vi "RT_TVA_2_boardcomp_DATA_vPXI.vi"(11 "TVA data":u8[](array[numeric])) -> (0 "TVA_Yaw [deg]":dbl, 1 "TVA_Pitch [deg]":dbl, 2 "Act 315 Angle \"Yaw\"":dbl(knob) scale=-3.0..3.0, 3 "Act 225 Angle \"Pitch\"":dbl(knob) scale=-3.0..3.0, 4 "CRC Check over Byte #10 to byte #84":bool, 5 "Control Variables (extra variables)":dbl[](array[numeric]), 6 "CRC Check over Byte #2 to Byte #7":bool)   [LabVIEW 2017]
panel:
  out "CRC data":u16 format="%x"
  out "CRC data comp":u16 format="%x"
  out "CRC addr":u16 format="%x"
  out "CRC addr comp":u16 format="%x"
  out "Roll DMARS [deg]":dbl
  out "Yaw DMARS [deg]":dbl
  out "Pitch DMARS [deg]":dbl
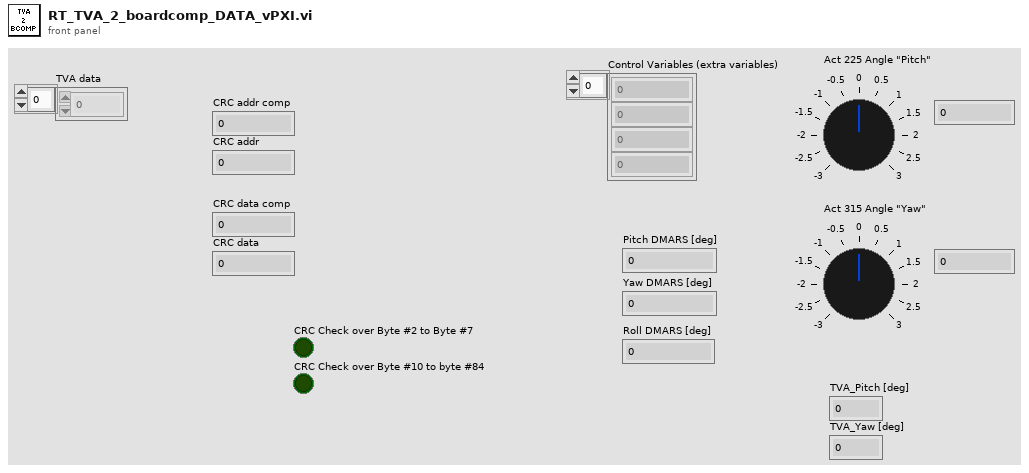
[diagram p1: front panel]
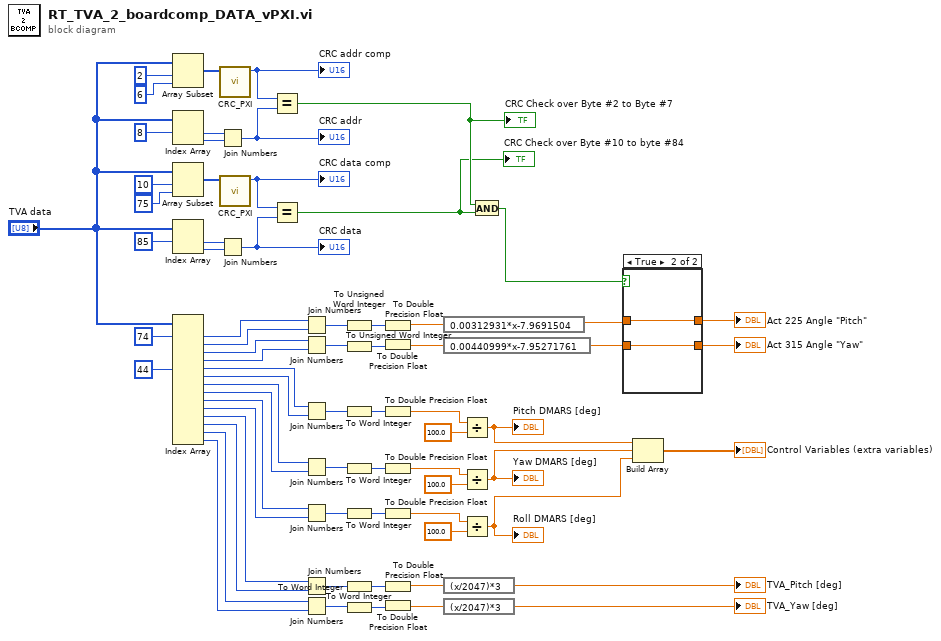
[diagram p0: block diagram]
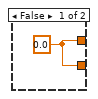
[diagram p2: hidden frame]
diagram:
  n1 = Array Subset(array="TVA data", index=2, length=6) -> (w37:u8[])
  n2 = Index Array(array="TVA data", index #1=8 ("index")) -> (element #1=w33:u8, element #2=w34:u8)  [unwired: 1 in]
  n3 = Array Subset(array="TVA data", index=10, length=75) -> (w27:u8[])
  n4 = Index Array(array="TVA data", index #1=85 ("index")) -> (element #1=w30:u8, element #2=w29:u8)  [unwired: 1 in]
  n5 = Index Array(array="TVA data", index #1=74 ("index"), index #5=44 ("index")) -> (element #1=w14:u8, element #2=w66:u8, element #3=w67:u8, element #4=w68:u8, element #5=w20:u8, element #6=w19:u8, element #7=w18:u8, element #8=w17:u8, element #9=w16:u8, element #10=w15:u8, element #11=w6:u8, element #12=w5:u8, element #13=w4:u8, element #14=w3:u8)  [unwired: 12 in]
  n6 = Join Numbers(hi=w33, lo=w34) -> ((hi.lo)=w32:u16)
  "CRC addr" <- w32
  n7 = Join Numbers(hi=w30, lo=w29) -> ((hi.lo)=w22:u16)
  "CRC data" <- w22
  n8 = call "CRC_PXI.vi"("Array"=w37) -> ("CRC"=w36:u16)  [unwired: 10 in]
  "CRC addr comp" <- w36
  n9 = call "CRC_PXI.vi"("Array"=w27) -> ("CRC"=w23:u16)  [unwired: 10 in]
  "CRC data comp" <- w23
  n10 = Equal?(x=w36, y=w32) -> (x = y?=w31:bool)
  "CRC Check over Byte #2 to Byte #7" <- w31
  n11 = Equal?(x=w23, y=w22) -> (x = y?=w24:bool)
  "CRC Check over Byte #10 to byte #84" <- w24
  n12 = Join Numbers(hi=w14, lo=w66) -> ((hi.lo)=w59:u16)
  n13 = Join Numbers(hi=w67, lo=w68) -> ((hi.lo)=w57:u16)
  n14 = Join Numbers(hi=w20, lo=w19) -> ((hi.lo)=w52:u16)
  n15 = Join Numbers(hi=w18, lo=w17) -> ((hi.lo)=w53:u16)
  n16 = Join Numbers(hi=w16, lo=w15) -> ((hi.lo)=w51:u16)
  n17 = Join Numbers(hi=w6, lo=w5) -> ((hi.lo)=w10:u16)
  n18 = Join Numbers(hi=w4, lo=w3) -> ((hi.lo)=w8:u16)
  n19 = To Unsigned Word Integer(number=w59) -> (unsigned 16bit integer=w58:u16)
  n20 = To Unsigned Word Integer(number=w57) -> (unsigned 16bit integer=w56:u16)
  n21 = To Word Integer(number=w52) -> (16bit integer=w55:i16)
  n22 = To Word Integer(number=w53) -> (16bit integer=w54:i16)
  n23 = To Word Integer(number=w51) -> (16bit integer=w50:i16)
  n24 = To Word Integer(number=w10) -> (16bit integer=w9:i16)
  n25 = To Word Integer(number=w8) -> (16bit integer=w7:i16)
  n26 = To Double Precision Float(number=w58) -> (double precision float=w70:dbl)
  n27 = To Double Precision Float(number=w56) -> (double precision float=w69:dbl)
  n28 = To Double Precision Float(number=w55) -> (double precision float=w48:dbl)
  n29 = To Double Precision Float(number=w54) -> (double precision float=w45:dbl)
  n30 = To Double Precision Float(number=w50) -> (double precision float=w44:dbl)
  n31 = To Double Precision Float(number=w9) -> (double precision float=w12:dbl)
  n32 = To Double Precision Float(number=w7) -> (double precision float=w11:dbl)
  n33 = expression code="0.00312931*x-7.9691504"(w70) -> (w61:dbl)
  n34 = expression code="0.00440999*x-7.95271761"(w69) -> (w60:dbl)
  n35 = expression code="(x/2047)*3"(w12) -> (→"TVA_Pitch [deg]":dbl)
  n36 = expression code="(x/2047)*3"(w11) -> (→"TVA_Yaw [deg]":dbl)
  n37 = Divide(x=w48, y=100.0) -> (x/y=w43:dbl)
  "Pitch DMARS [deg]" <- w43
  n38 = Divide(x=w45, y=100.0) -> (x/y=w42:dbl)
  "Yaw DMARS [deg]" <- w42
  n39 = Divide(x=w44, y=100.0) -> (x/y=w41:dbl)
  "Roll DMARS [deg]" <- w41
  n40 = And(x=w31, y=w24) -> (x .and. y?=w64:bool)
  n41 = case shown="True" w64 {
    tunnel: [w71 w73] -> w63
    tunnel: [w71 w72] -> w62
    tunnel: w61 -> [_ w73]
    tunnel: w60 -> [_ w72]
    frame False {
      w71 = 0.0
    }
    frame True {
    }
  }
  "Act 315 Angle \"Yaw\"" <- w62
  "Act 225 Angle \"Pitch\"" <- w63
  n42 = Build Array(w43, w42, w41) -> (→"Control Variables (extra variables)":dbl[])
